vi "Simple TCP - Server.vi"() -> ()   [LabVIEW 2013]
doc: "Demonstrates how to set up a basic TCP connection, send data to the specified port once a connection has been established, and terminate the connection once the data has been sent. This VI is designed to stop if the TCP connection is terminated. The data sent in this example is an array of random numbers."
panel:
  out "Data from Client":dbl
  in  "Data to Client":dbl=12.0
  in  "Stop":bool
  # "Overview: Implements a simple TCP server that can send data to a client\nInstructions:\n1. Run the VI.\n2. Deploy the Veristand project containing TCPIP Custom Device\n3. If you undeploy the TCPIP Custom Device, this VI will stop automatically."
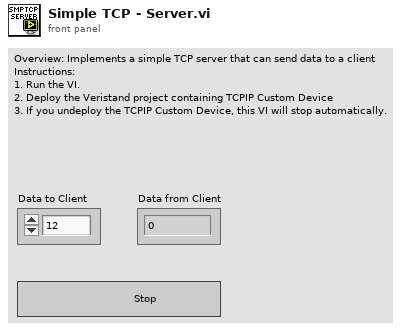
[diagram p1: front panel]
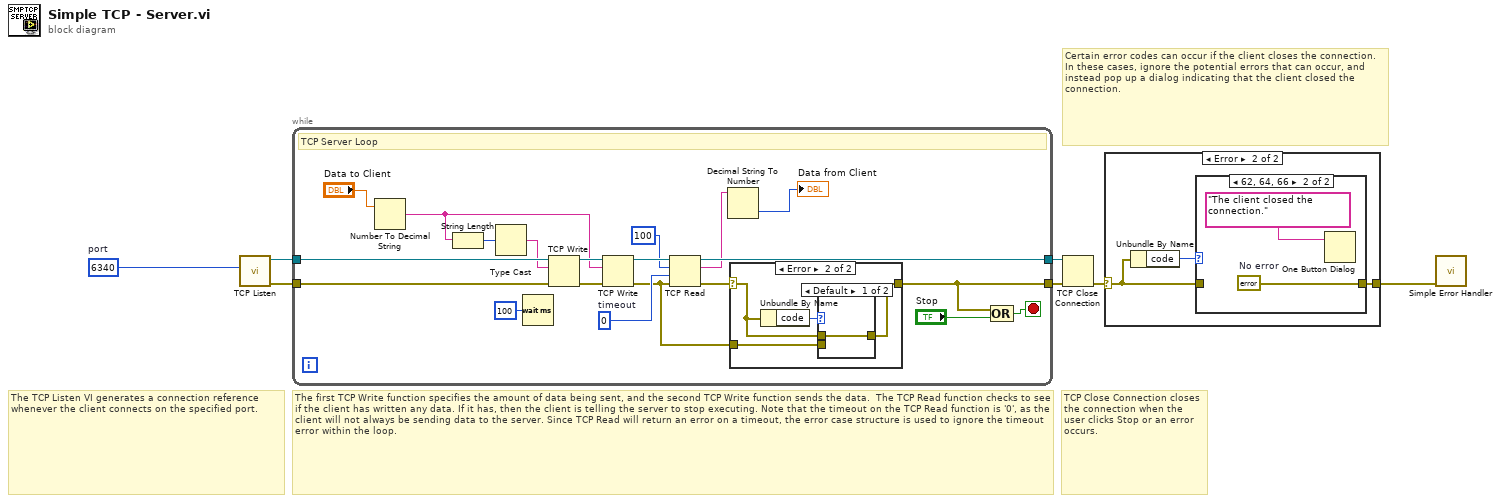
[diagram p0: block diagram]
diagram:
  w1 = u16 6340  # port
  # "TCP Close Connection closes the connection when the user clicks Stop or an error occurs."
  # "The TCP Listen VI generates a connection reference whenever the client connects on the specified port."
  # "Certain error codes can occur if the client closes the connection. In these cases, ignore the potential errors that can occur, and instead pop up a dialog indicating that the client closed the connection."
  # "The first TCP Write function specifies the amount of data being sent, and the second TCP Write function sends the data.  The TCP Read function checks to see if the client has written any data. If it has, then the client is telling the server to stop executing. Note that the timeout on the TCP Read function is '0', as the client will not always be sending data to the server. Since TCP Read will return an error on a timeout, the error case structure is used to ignore the timeout error within the loop."
  n1 = call <vilib>:"TCP Listen.vi"("port"=w1) -> ("error out"=w2:errorcluster, "connection ID"=w3:refnum<k5>)  [unwired: 6 in, 3 out]
  n2 = while {
    tunnel: [w14] -> w6
    tunnel: [w17] -> w7
    tunnel: w3 -> [w27]
    tunnel: w2 -> [w20]
    stop <- w21 stop-if-true
    w16 = 0  # timeout
    # "TCP Server Loop"
    n3 = Number To Decimal String(number="Data to Client") -> (decimal integer string=w10:string)  [unwired: 1 in]
    n4 = String Length(string=w10) -> (length=w24:i32)
    n5 = Type Cast(x=w24) -> (*(type *) &x=w23:string)  [unwired: 1 out]
    n6 = Wait (ms)(milliseconds to wait=u32 100) -> ()  [unwired: 1 out]
    n7 = TCP Write(connection ID=w27, data in=w23, error in (no error)=w20) -> (connection ID out=w26:refnum<k5>, error out=w25:errorcluster)  [unwired: 2 out]
    n8 = TCP Write(connection ID=w26, data in=w10, error in (no error)=w25) -> (connection ID out=w18:refnum<k5>, error out=w13:errorcluster)  [unwired: 2 out]
    n9 = TCP Read(connection ID=w18, bytes to read=100, error in (no error)=w13, 9:w16) -> (connection ID out=w17:refnum<k5>, data out=w9:string, error out=w15:errorcluster)  [unwired: 1 out]
    n10 = Decimal String To Number(string=w9) -> (number=→"Data from Client":i32)  [unwired: 2 in, 1 out]
    n11 = case shown="Error" w15 {
      selector: w15 -> [w28 w31]
      tunnel: [w28 w29] -> w14
      tunnel: w13 -> [_ w30]
      frame No Error {
      }
      frame Error {
        n12 = Unbundle By Name(w31) -> ("code"=w32:i32)
        n13 = case shown="Default" w32 {
          tunnel: w31 -> [w33 _]
          tunnel: w30 -> [_ w34]
          tunnel: [w33 w34] -> w29
          frame Default {
          }
          frame 56 {
          }
        }
      }
    }
    n14 = Compound Arithmetic op=OR(w14, "Stop") -> (w21:bool)
  }
  n15 = TCP Close Connection(connection ID=w7, error in (no error)=w6) -> (error out=w5:errorcluster)  [unwired: 2 out]
  n16 = case shown="Error" w5 {
    selector: w5 -> [w35 w37]
    tunnel: [w35 w36] -> w4
    frame No Error {
    }
    frame Error {
      n17 = Unbundle By Name(w37) -> ("code"=w38:i32)
      n18 = case shown="62, 64, 66" w38 {
        tunnel: w37 -> [w39 _]
        tunnel: [w39 w41] -> w36
        frame Default {
        }
        frame 62, 64, 66 {
          w41 = errorcluster {"status"=FALSE, "code"=0, "source"=""}  # No error
          n19 = One Button Dialog(message="The client closed the connection." ("Client Closed")) -> ()  [unwired: 1 in, 1 out]
        }
      }
    }
  }
  n20 = call <vilib>:"Simple Error Handler.vi"("error in (no error)"=w4) -> ()  [unwired: 1 in, 8 out]
